vi "generate table.vi"(4 "Slaves to Enable Diagnostics":refnum<vi>, 6 "Available Slaves":refnum<vi>, 7 "table":T1, 8 "error in":errorcluster, 10 "engine configuration in":refnum<class "engine configuration.lvclass">, 11 "Profibus Module configuration in":refnum<class "Profibus Module configuration.lvclass">) -> (0 "error out":errorcluster)   [LabVIEW 2013, in "Profibus Module editor node.lvclass"]
uses:
  Profibus Module editor node.lvclass
  table reference.ctl
  configuration/Profibus Module configuration.lvclass
  <vilib>/NI/Module Execution Interface/Engine Configuration/engine configuration.lvclass
  <vilib>/NI/Configuration Framework/serializable configuration/NISE_CEF_serializable configuration.lvclass/NISE_CEF_serializable configuration.ctl
  <vilib>/NI/Configuration Framework/serializable configuration/NISE_CEF_serializable configuration.lvclass
  configuration/Profibus Module configuration.lvclass/Profibus Module configuration.ctl
  table line.ctl
  channel/Profibus channel.lvclass
  channel/Profibus channel.lvclass/Profibus channel.ctl
  <vilib>/NI/Tag Bus/tag/tag descriptor.lvclass/tag descriptor.ctl
  channel/Read slave.vi
  <vilib>/NI/Tag Bus/tag/read tag name.vi
  <vilib>/NI/Configuration Framework/serializable configuration/Read UID.vi
  configuration/Read slave diagnostics.vi
  <vilib>/NI/Tag Bus Module Framework/channel/TBM channel.lvclass
  <vilib>/NI/Tag Bus/tag/tag descriptor.lvclass
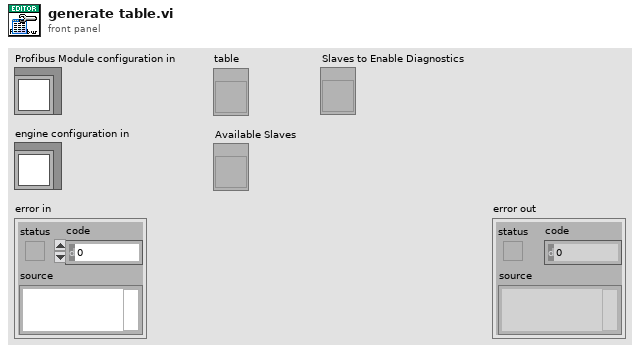
[diagram p1: front panel]
types:
  T1 = typedef "Profibus Module editor node.lvclass/table reference.ctl" = refnum<vi>
  T2 = typedef "Profibus Module configuration.lvclass/slave diagnostic configuration.ctl" = cluster{"slave":i8, "report":bool, "channel":refnum<class "TBM channel.lvclass">, "error specs":T3[]}
  T3 = typedef "Profibus Module configuration.lvclass/error throw specification.ctl" = cluster{"byte":i32, "bit":i32, "inverted?":bool, "error":i32}
  T4 = typedef "Profibus Module editor node.lvclass/table line.ctl" = cluster{"profchan":refnum<class "Profibus channel.lvclass">, "tag name":string}
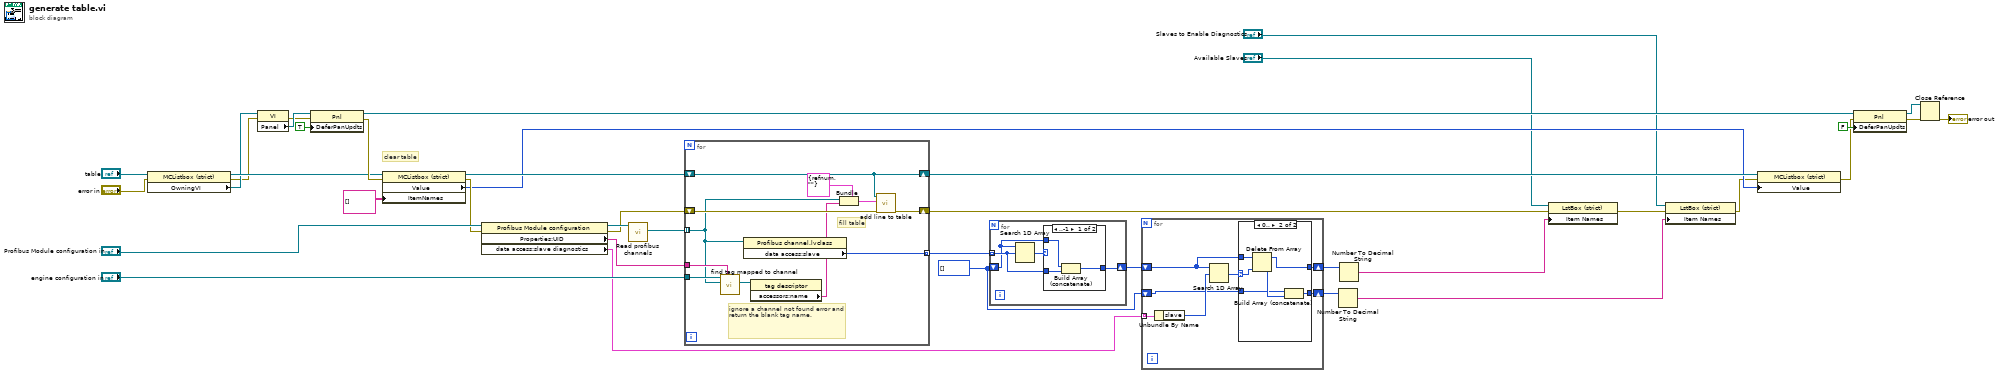
[diagram p0: block diagram]
diagram:
  w9 = i8[] []
  # "clear table"
  n1 = property class="MCListbox (strict)"(reference="table", error in="error in") -> (reference out=w18:T1, error out=w15:errorcluster, "OwningVI"=w16:refnum<vi>)
  n2 = property class="VI"(reference=w16, error in=w15) -> (error out=w24:errorcluster, "Panel"=w25:refnum<vi>)  [unwired: 1 out]
  n3 = property class="Pnl"(reference=w25, error in=w24, "DeferPanUpdts"=TRUE ("Defer Panel Updates")) -> (reference out=w21:refnum<vi>, error out=w23:errorcluster)
  n4 = property class="MCListbox (strict)"(reference=w18, error in=w23, "ItemNames"=string[][] [] ("Item Names")) -> (reference out=w37:T1, error out=w32:errorcluster, "Value"=w27:i32)
  n5 = property class="Profibus Module configuration"(reference="Profibus Module configuration in", error in=w32) -> (reference out=w34:refnum<class "Profibus Module configuration.lvclass">, error out=w31:errorcluster, "Properties:UID"=w33:string, "data access:slave diagnostics"=w10:T2[])
  n6 = call "Read profibus channels.vi"("Profibus Module configuration in"=w34) -> ("channels"=w38:refnum<class "Profibus channel.lvclass">[])  [unwired: 8 in, 2 out]
  n7 = for {
    shift-right: [w50] -> w28
    shift-left: w31 -> [w47]
    tunnel: w38 -> [w41] mode=indexing
    tunnel: "engine configuration in" -> [w46]
    tunnel: w33 -> [w45]
    shift-right: [w42] -> w29
    shift-left: w37 -> [w42]
    tunnel: [w40] -> w12 mode=indexing
    # "ignore a channel not found error and return the blank tag name."
    # "fill table"
    n8 = call <vilib>:"find tag mapped to channel.vi"("owner"=w45, "channel"=w41, "engine configuration in"=w46) -> ("tag"=w44:refnum<class "tag descriptor.lvclass">)  [unwired: 6 in, 2 out]
    n9 = property class="Profibus channel.lvclass"(reference=w41) -> ("data access:slave"=w40:i8)  [unwired: 1 in, 2 out]
    n10 = property class="tag descriptor"(reference=w44) -> ("accessors:name"=w43:string)  [unwired: 1 in, 2 out]
    n11 = Bundle(cluster=T4 {"profchan"=refnum, "tag name"=""} ("line"), "profchan"=w41, "tag name"=w43) -> (w48:T4)
    n12 = call "add line to table.vi"("error in"=w47, "line"=w48, "operations table"=w42) -> ("error out"=w50:errorcluster)  [unwired: 8 in]
  }
  n13 = for {
    tunnel: w12 -> [w53] mode=indexing
    shift-right: [w52] -> w11
    shift-left: w9 -> [w51]
    n14 = Search 1D Array(1D array=w51, element=w53) -> (index of element=w54:i32)  [unwired: 1 in]
    n15 = case shown="..-1" w54 {
      tunnel: w53 -> [w57 _]
      tunnel: [w56 w58] -> w52
      tunnel: w51 -> [w55 w58]
      frame ..-1 {
        n16 = Build Array (concatenate)(w55, w57) -> (w56:i8[])
      }
      frame 0.. {
      }
    }
  }
  n17 = for {
    shift-right: [w61] -> w4
    shift-left: w11 -> [w62]
    tunnel: w10 -> [w65] mode=indexing
    shift-right: [w60] -> w3
    shift-left: w9 -> [w59]
    n18 = Unbundle By Name(w65) -> ("slave"=w64:i8)
    n19 = Search 1D Array(1D array=w62, element=w64) -> (index of element=w63:i32)  [unwired: 1 in]
    n20 = case shown="0.." w63 {
      selector: w63 -> [_ w72]
      tunnel: w62 -> [w67 w73]
      tunnel: [w67 w71] -> w61
      tunnel: [w66 w69] -> w60
      tunnel: w59 -> [w66 w68]
      frame ..-1 {
      }
      frame 0.. {
        n21 = Delete From Array(array=w73, index=w72) -> (deleted portion=w70:i8, array with subset deleted=w71:i8[])  [unwired: 1 in]
        n22 = Build Array (concatenate)(w68, w70) -> (w69:i8[])
      }
    }
  }
  n23 = Number To Decimal String(number=w3) -> (decimal integer string=w1:string[])  [unwired: 1 in]
  n24 = Number To Decimal String(number=w4) -> (decimal integer string=w2:string[])  [unwired: 1 in]
  n25 = property class="LstBox (strict)"(reference="Available Slaves", error in=w28, "Item Names"=w2) -> (error out=w8:errorcluster)  [unwired: 1 out]
  n26 = property class="LstBox (strict)"(reference="Slaves to Enable Diagnostics", error in=w8, "Item Names"=w1) -> (error out=w7:errorcluster)  [unwired: 1 out]
  n27 = property class="MCListbox (strict)"(reference=w29, error in=w7, "Value"=w27) -> (error out=w20:errorcluster)  [unwired: 1 out]
  n28 = property class="Pnl"(reference=w21, error in=w20, "DeferPanUpdts"=FALSE ("Defer Panel Updates")) -> (reference out=w13:refnum<vi>, error out=w19:errorcluster)
  n29 = Close Reference(reference=w13, error in (no error)=w19) -> (error out=→"error out":errorcluster)
